vi "paths.get.vi"(11 "manager_daemon in":refnum<class "manager_daemon.lvclass">) -> (2 "paths":T1, 3 "manager_daemon out":refnum<class "manager_daemon.lvclass">)   [LabVIEW 2024, in "manager_daemon.lvclass"]
uses:
  manager_daemon.lvclass
  manager_daemon.lvclass/manager_daemon.ctl
  type_defs/paths--cluster.ctl
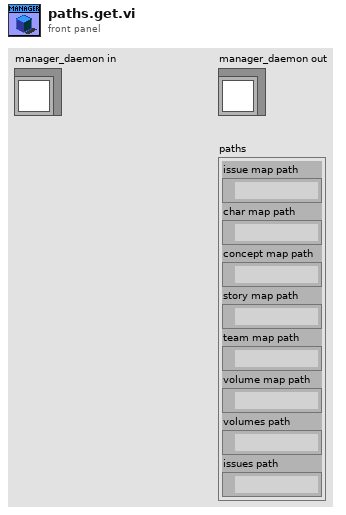
[diagram p1: front panel]
types:
  T1 = typedef "manager_daemon.lvclass/paths--cluster.ctl" = cluster{"issue map path":path, "char map path":path, "concept map path":path, "story map path":path, "team map path":path, "volume map path":path, "volumes path":path, "issues path":path}
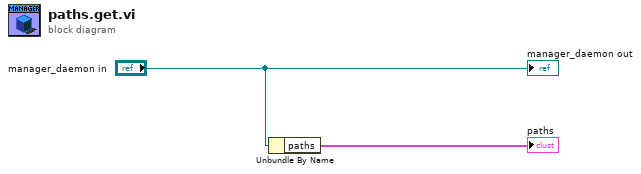
[diagram p0: block diagram]
diagram:
  n1 = Unbundle By Name("manager_daemon in") -> ("paths"=→"paths":T1)
  "manager_daemon out" <- "manager_daemon in"
